vi "DAQ_change_plot_display.vi"(3 "error in":errorcluster, 4 "WFChart Refnum":refnum<vi>, 5 "selection":u16) -> (0 "error out":errorcluster)   [LabVIEW 2015]
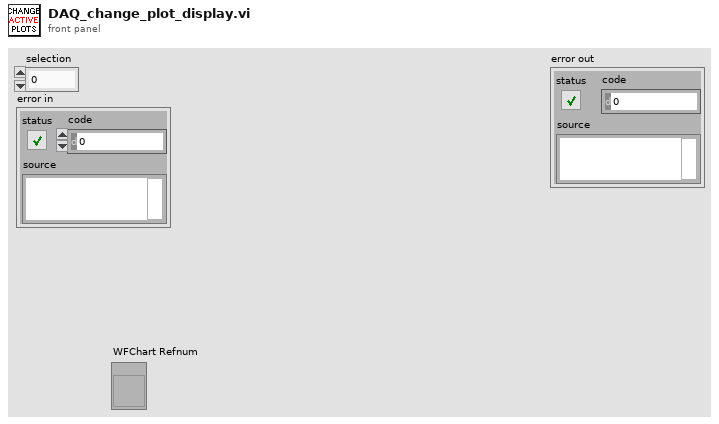
[diagram p1: front panel]
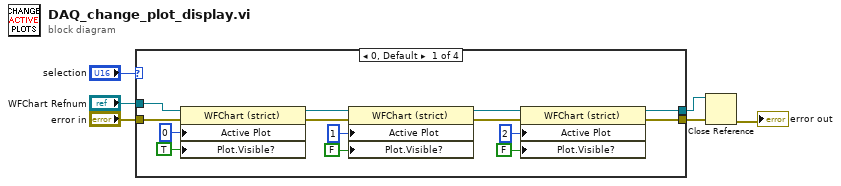
[diagram p0: block diagram]
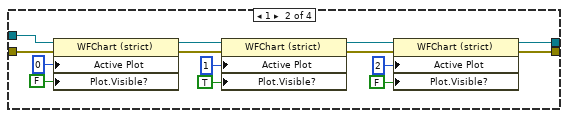
[diagram p2: hidden frame]
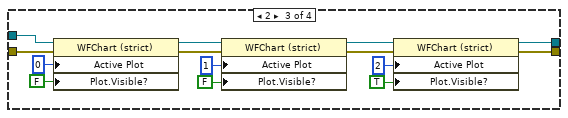
[diagram p3: hidden frame]
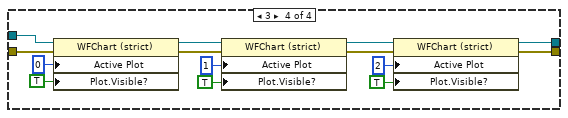
[diagram p4: hidden frame]
diagram:
  n1 = case shown="0, Default" "selection" {
    tunnel: "error in" -> [w8 w22 w36 w50]
    tunnel: "WFChart Refnum" -> [w20 w34 w48 w62]
    tunnel: [w9 w23 w37 w51] -> w3
    tunnel: [w7 w21 w35 w49] -> w2
    frame 0, Default {
      n2 = property class="WFChart (strict)"(reference=w20, error in=w8, "Active Plot"=u32 0, "Plot.Visible?"=TRUE ("Plot.Visible")) -> (reference out=w15:refnum<vi>, error out=w14:errorcluster)
      n3 = property class="WFChart (strict)"(reference=w15, error in=w14, "Active Plot"=u32 1, "Plot.Visible?"=FALSE ("Plot.Visible")) -> (reference out=w11:refnum<vi>, error out=w10:errorcluster)
      n4 = property class="WFChart (strict)"(reference=w11, error in=w10, "Active Plot"=u32 2, "Plot.Visible?"=FALSE ("Plot.Visible")) -> (reference out=w7:refnum<vi>, error out=w9:errorcluster)
    }
    frame 1 {
      n5 = property class="WFChart (strict)"(reference=w34, error in=w22, "Active Plot"=u32 0, "Plot.Visible?"=FALSE ("Plot.Visible")) -> (reference out=w29:refnum<vi>, error out=w28:errorcluster)
      n6 = property class="WFChart (strict)"(reference=w29, error in=w28, "Active Plot"=u32 1, "Plot.Visible?"=TRUE ("Plot.Visible")) -> (reference out=w25:refnum<vi>, error out=w24:errorcluster)
      n7 = property class="WFChart (strict)"(reference=w25, error in=w24, "Active Plot"=u32 2, "Plot.Visible?"=FALSE ("Plot.Visible")) -> (reference out=w21:refnum<vi>, error out=w23:errorcluster)
    }
    frame 2 {
      n8 = property class="WFChart (strict)"(reference=w48, error in=w36, "Active Plot"=u32 0, "Plot.Visible?"=FALSE ("Plot.Visible")) -> (reference out=w43:refnum<vi>, error out=w42:errorcluster)
      n9 = property class="WFChart (strict)"(reference=w43, error in=w42, "Active Plot"=u32 1, "Plot.Visible?"=FALSE ("Plot.Visible")) -> (reference out=w39:refnum<vi>, error out=w38:errorcluster)
      n10 = property class="WFChart (strict)"(reference=w39, error in=w38, "Active Plot"=u32 2, "Plot.Visible?"=TRUE ("Plot.Visible")) -> (reference out=w35:refnum<vi>, error out=w37:errorcluster)
    }
    frame 3 {
      n11 = property class="WFChart (strict)"(reference=w62, error in=w50, "Active Plot"=u32 0, "Plot.Visible?"=TRUE ("Plot.Visible")) -> (reference out=w57:refnum<vi>, error out=w56:errorcluster)
      n12 = property class="WFChart (strict)"(reference=w57, error in=w56, "Active Plot"=u32 1, "Plot.Visible?"=TRUE ("Plot.Visible")) -> (reference out=w53:refnum<vi>, error out=w52:errorcluster)
      n13 = property class="WFChart (strict)"(reference=w53, error in=w52, "Active Plot"=u32 2, "Plot.Visible?"=TRUE ("Plot.Visible")) -> (reference out=w49:refnum<vi>, error out=w51:errorcluster)
    }
  }
  n14 = Close Reference(reference=w2, error in (no error)=w3) -> (error out=→"error out":errorcluster)
